vi "Main.vi"(7 "ConcreteActor":refnum<class "ConcreteActor.lvclass">, 10 "ErrorQueue":refnum<queue>, 11 "PreSetupQueue":refnum<queue>) -> (4 "Error":errorcluster, 5 "ConcreteActor":refnum<class "ConcreteActor.lvclass">)   [LabVIEW 2020, in "_Template.lvlib" / "ActorTemplate.lvlib" / "{{Name}}.lvlib" / "ConcreteActor.lvclass"]
uses:
  ConcreteActor.lvclass
  ConcreteActor.lvclass/ConcreteActor.ctl
  C:/jettl-harness/repos/jettl/src/jettl/jettl/Actor/Actor.lvclass
  jettl/jettl/jettl.lvlib
  jettl/jettl/PreSetup.ctl
panel:
  # "This panel can be extended with controls and indicators, though do not modify the conn pane."
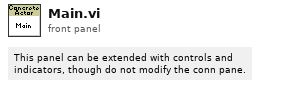
[diagram p1: front panel]
types:
  T1 = cluster{"EventRegistrationRef":refnum<event-registration>}
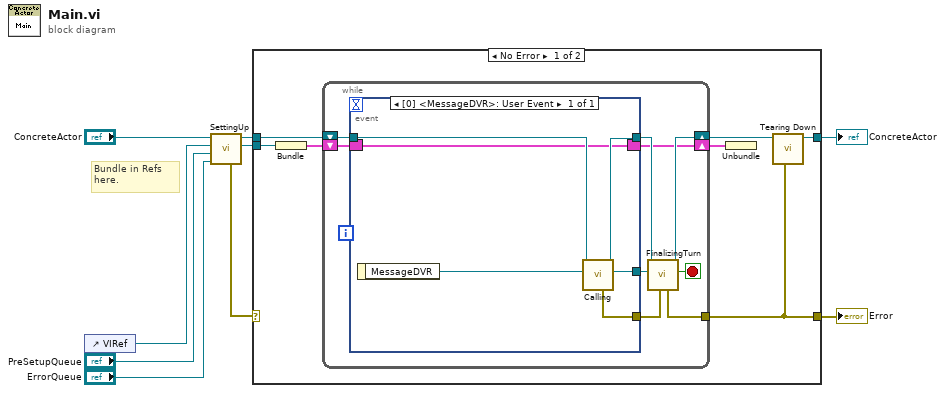
[diagram p0: block diagram]
diagram:
  # "Bundle in Refs here."
  n1 = control-ref of="VIRef"() -> (w4:refnum<vi>)
  n2 = call "SettingUp.vi"("ErrorQueue"="ErrorQueue", "PreSetup"="PreSetupQueue", "VIRef"=w4, "Actor"="ConcreteActor") -> ("EventRegistrationRef"=w7:refnum<event-registration>, "Actor"=w5:refnum<class "ConcreteActor.lvclass">, "Error"=w3:errorcluster)  [unwired: 5 in]
  n3 = case shown="No Error" w3 {
    selector: w3 -> [_ w32]
    tunnel: [w14 w33] -> w9
    tunnel: w5 -> [w16 w33]
    tunnel: [w13 w32] -> w8
    tunnel: w7 -> [w12 _]
    frame No Error {
      n4 = Bundle("EventRegistrationRef"=w12) -> (w11:T1)  [unwired: 1 in]
      n5 = while {
        shift-right: [w19] -> w15
        shift-left: w16 -> [w25]
        tunnel: [w22] -> w13
        shift-right: [w17] -> w10
        shift-left: w11 -> [w18]
        stop <- w24 stop-if-true
        n6 = event shown="[0] <MessageDVR>: User Event" {
          selector: w18 -> [w26]
          dyn-events: [w26] -> w17
          timeout: _ -> [_]
          tunnel: w25 -> [w30]
          tunnel: [w29] -> w20
          tunnel: [w28] -> w23
          tunnel: [w27] -> w21
          event User Event {
            n7 = event-data() -> ("MessageDVR"=w31:refnum<data-value>)  [unwired: 1 in]
            n8 = call "Calling.vi"("MessageDVR"=w31, "Actor"=w30) -> ("Message"=w27:refnum<class "Message.lvclass">, "Actor"=w29:refnum<class "ConcreteActor.lvclass">, "Error"=w28:errorcluster)  [unwired: 7 in]
          }
        }
        n9 = call "FinalizingTurn.vi"("Error"=w23, "Message"=w21, "Actor"=w20) -> ("ProceedToTearingDown"=w24:bool, "Actor"=w19:refnum<class "ConcreteActor.lvclass">, "Error"=w22:errorcluster)  [unwired: 6 in]
      }
      n10 = Unbundle(w10) -> ()  [unwired: 1 out]
      n11 = call "Tearing Down.vi"("Error"=w13, "Actor"=w15) -> ("Actor"=w14:refnum<class "ConcreteActor.lvclass">)  [unwired: 9 in]
    }
    frame Error {
    }
  }
  "ConcreteActor" <- w9
  "Error" <- w8
